vi "VIPM_Filter Paths.vi"(11 "Unfiltered map in":map{string, string[]}(c390)) -> (3 "Filtered map out":map{string, string[]}(c390))   [LabVIEW 2019, in "Project.Dependencies Finder.lvlib" / "Dependency Source_VIPM.lvclass"]
doc: "If user.lib, vi.lib or instr.lib are in the map only these will be allowed to remain."
uses:
  Dependency Source_VIPM.lvclass
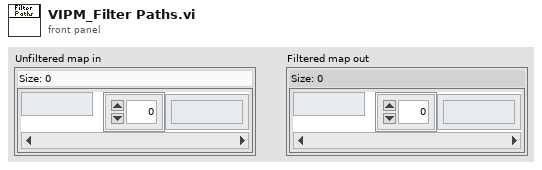
[diagram p1: front panel]
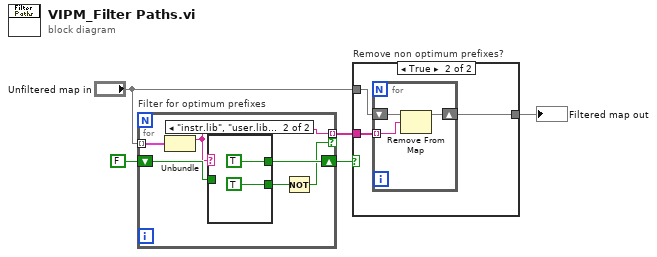
[diagram p0: block diagram]
diagram:
  n1 = for "Filter for optimum prefixes" {
    tunnel: "Unfiltered map in" -> [w11] mode=indexing
    shift-right: [w9] -> w2
    shift-left: FALSE -> [w10]
    tunnel: [w7] -> w5 mode=indexing if=w6
    n2 = Unbundle(w11) -> ("key"=w7:string)  [unwired: 1 out]
    n3 = case shown="\"instr.lib\", \"user.lib\", \"vi.lib\"" w7 {
      tunnel: w10 -> [w12 _]
      tunnel: [w12 TRUE] -> w9
      tunnel: [_ TRUE] -> w8
      frame Default {
      }
      frame "instr.lib", "user.lib", "vi.lib" {
      }
    }
    n4 = Not(x=w8) -> (.not. x?=w6:bool)
  }
  n5 = case "Remove non optimum prefixes?" shown="True" w2 {
    tunnel: [w15 w17] -> w4
    tunnel: "Unfiltered map in" -> [w15 w18]
    tunnel: w5 -> [_ w16]
    frame False {
    }
    frame True {
      n6 = for {
        tunnel: w16 -> [w19] mode=indexing
        shift-right: [w20] -> w17
        shift-left: w18 -> [w21]
        n7 = Remove From Map(10:w19, 11:w21) -> (3:w20:map{string, string[]})  [unwired: 2 out]
      }
    }
  }
  "Filtered map out" <- w4
